vi "detect_bool_change.vi"(10 "Boolean in":bool, 11 "Boolean 3":bool) -> (2 "x > y?":bool)   [LabVIEW 2017]
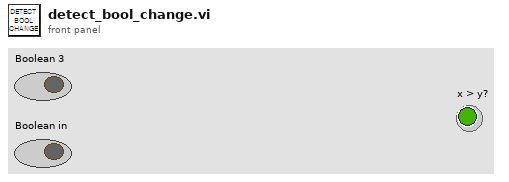
[diagram p1: front panel]
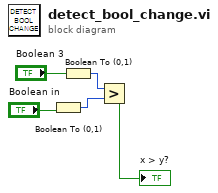
[diagram p0: block diagram]
diagram:
  n1 = Boolean To (0,1)(Boolean="Boolean in") -> (0, 1=w5:i16)
  n2 = Boolean To (0,1)(Boolean="Boolean 3") -> (0, 1=w4:i16)
  n3 = Greater?(x=w4, y=w5) -> (0:→"x > y?":bool)
